vi "Test-XBox Controller-Request Updates.vi"() -> ()   [LabVIEW 2014, in "Comp XBox One Controller.lvlib"]
uses:
  Comp XBox One Controller.lvlib
  Robot Actor Framework/Trace/Trace Controller Class/Config.ctl
  Comp Motors with Encoders/Comp Motors with Encoders Class/Encoder Config.ctl
  Comp Motors with Encoders/Comp Motors with Encoders Class/Motor Controller Config.ctl
  Robot/Motor with Encoders/Motors with Encoders Class/Motors with Encoders Config.ctl
  Robot/Motor with Encoders/Motors with Encoders Class/Motors with Encoders State.ctl
  Comp Motors with Brake/Comp Motors with Brake Class/Comp Motors with Brake Config.ctl
  <vilib>/Rock Robotics/WPI/Solenoid/WPI_SolenoidChannel.ctl
  Comp Trace Controller/Comp Trace Controller Class/Comp Trace Controller.lvclass
  Comp Pressure/Comp Pressure Class/Comp Pressure.lvclass
  Comp Motors with Encoders/Receive Updates from Motors with Encoders Class/Receive Updates from Motors with Encoders.lvclass
  Comp Motors with Brake/Comp Motors with Brake Class/Comp Motors with Brake.lvclass
  <vilib>/Rock Robotics/WPI/DriverStation/WPI_DriverStationRobotMode2.ctl
  Comp Motors with Encoders/Receive Updates from Motors with Encoders Messages/Receive Update from Motors Msg/Receive Update from Motors Msg.lvclass
  Robot/Motor with Encoders/Motors with Encoders Messages/Request Motors with Encoders State Msg/Request Motors with Encoders State Msg.lvclass/Request Motors with Encoders State Msg.ctl
  <vilib>/ActorFramework/Message Enqueuer/Message Enqueuer.lvclass/Message Enqueuer.ctl
  Robot/Motor with Encoders/Motors with Encoders Messages/Set Rate (Percent) Msg/Set Rate (Percent) Msg.lvclass/Set Rate (Percent) Msg.ctl
  <vilib>/ActorFramework/Message Enqueuer/Enqueue.vi
  <vilib>/ActorFramework/Message Priority Queue/Priority Enqueue.vi
  Robot/Motor with Encoders/Motors with Encoders Messages/Request Motors with Encoders State Msg/Request Motors with Encoders State Msg.lvclass
  Robot/Motor with Encoders/Motors with Encoders Messages/Set Rate (Percent) Msg/Set Rate (Percent) Msg.lvclass
  <vilib>/ActorFramework/Stop Msg/Stop Msg.lvclass
  <vilib>/ActorFramework/Actor/Actor.lvclass
  Robot Actor Framework/Trace/Trace Controller Class/Trace Controller.lvclass
  Comp Motors with Encoders/Comp Motors with Encoders Class/Comp Motors with Encoders.lvclass
  Robot/Motor with Encoders/Motors with Encoders Class/Motors with Encoders.lvclass
panel:
  in  "Rate":dbl=0.5
  in  "Direction":enum32{"Up", "Hold", "Down"}(radio)
  in  "Comp Motors with Brake Config":T1={"Brake Channel"=enum."Solenoid 6", "Pneumatics CAN ID"=3}
  in  "Motors with Encoder State":T3={"Forward Switch"=FALSE, "Reverse Switch"=FALSE, "Measured RPM"=0.0, "Distance (in)"=0.0, "Setpoint RPM"=0.0, "Encoder Count"=0, "Home Count"=0, "Config"={"Counts  Per Revolution"=0, "Invert Encoder Direction"=FALSE, "Diameter of Revolution"=0.0, "Max RPM"=0.0, "Encoder Control"=TRUE}}
  in  "Motors with Encoders Config":T4={"Counts  Per Revolution"=256, "Invert Encoder Direction"=FALSE, "Diameter of Revolution"=1.5, "Max RPM"=500.0, "Encoder Control"=TRUE}
  in  "Slave Motor Controller Configs":T5[](array[typedef])
  in  "Master Motor Controller Config":T5={"Device Number"=7, "Invert Motor"=FALSE}
  in  "Encoder Config":T6={"P"=1.0, "D"=0.0, "F"=0.01, "I"=0.01, "Reverse Feedback Sensor"=FALSE, "Encoder Codes Per Rev"=256}
  in  "Test Loop":u32=75
  out "Enable Tele":bool caption="Enabled Teleop"
  in  "Stop Test Loop 1":bool=TRUE
  in  "Finish Test":bool=TRUE
  in  "Start Test":bool=TRUE
  in  "Trace Controller Config":T7={"Folder Pattern"="/media/sd%s1", "Starting Letter Position"=1, "Min Free Space (MB)"=50.0, "Max Folders to Check"=10, "Trace Level"=enum."Debug"} {"Min Free Space (MB)" format="%#_13g"}
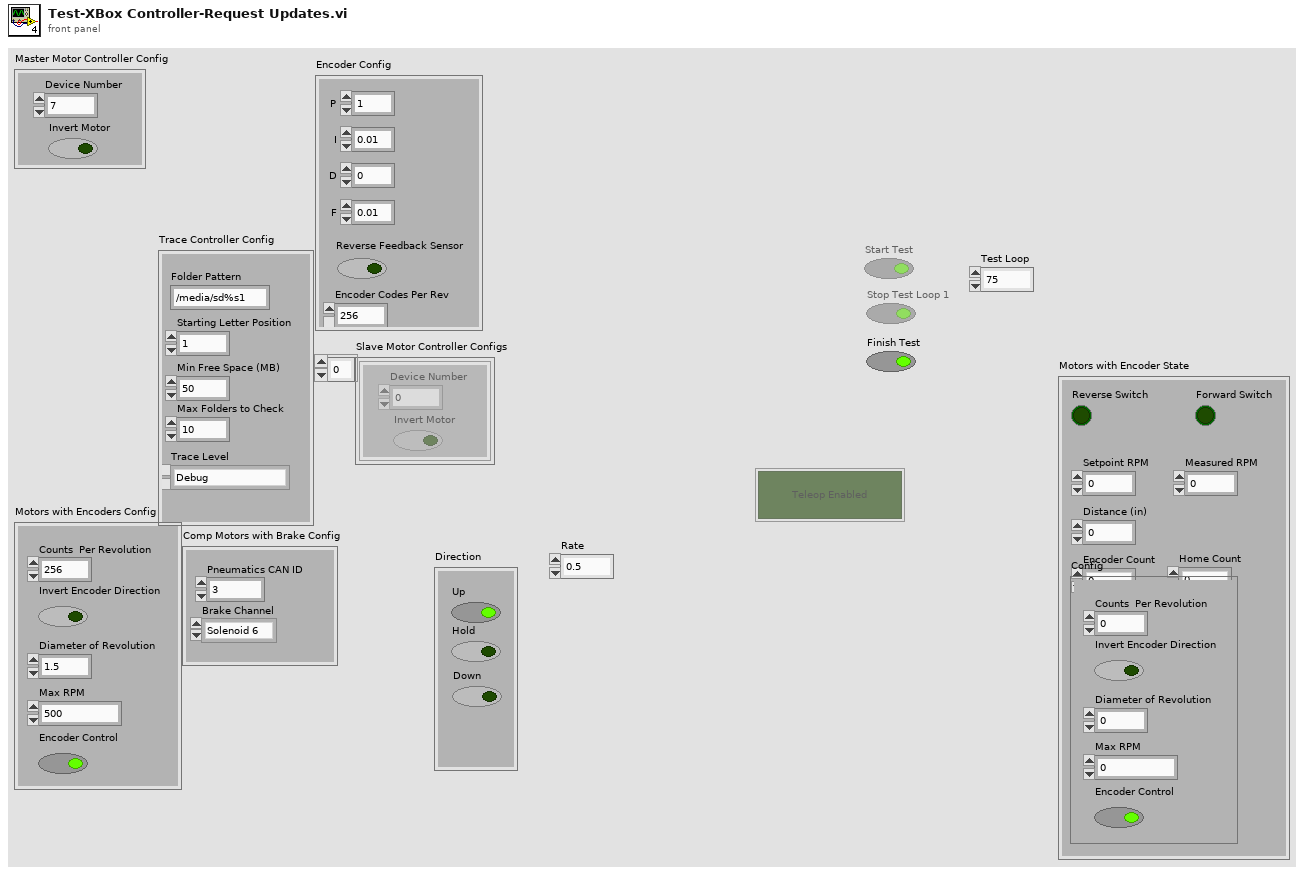
[diagram p1: front panel]
types:
  T1 = typedef "Comp Motors with Brake.lvlib/Comp Motors with Brake.lvclass/Comp Motors with Brake Config.ctl" = cluster{"Brake Channel":T2, "Pneumatics CAN ID":u8}
  T2 = typedef "WPI_SolenoidChannel.ctl" = enum8{"Solenoid 0", "Solenoid 1", "Solenoid 2", "Solenoid 3", "Solenoid 4", "Solenoid 5", "Solenoid 6", "Solenoid 7", "Invalid"}
  T3 = typedef "Motors with Encoders.lvlib/Motors with Encoders.lvclass/Motors with Encoders State.ctl" = cluster{"Forward Switch":bool, "Reverse Switch":bool, "Measured RPM":dbl, "Distance (in)":dbl, "Setpoint RPM":dbl, "Encoder Count":i64, "Home Count":i64, "Config":T4}
  T4 = typedef "Motors with Encoders.lvlib/Motors with Encoders.lvclass/Motors with Encoders Config.ctl" = cluster{"Counts  Per Revolution":u32, "Invert Encoder Direction":bool, "Diameter of Revolution":dbl, "Max RPM":dbl, "Encoder Control":bool}
  T5 = typedef "Comp Motors with Encoders.lvlib/Comp Motors with Encoders.lvclass/Motor Controller Config.ctl" = cluster{"Device Number":u8, "Invert Motor":bool}
  T6 = typedef "Comp Motors with Encoders.lvlib/Comp Motors with Encoders.lvclass/Encoder Config.ctl" = cluster{"P":dbl, "D":dbl, "F":dbl, "I":dbl, "Reverse Feedback Sensor":bool, "Encoder Codes Per Rev":u16}
  T7 = typedef "Robot Actor Framework.lvlib/Trace.lvlib/Trace Controller.lvclass/Config.ctl" = cluster{"Folder Pattern":string, "Starting Letter Position":i32, "Min Free Space (MB)":dbl, "Max Folders to Check":u32, "Trace Level":enum16{"Critical", "Error", "Warning", "Informational", "Debug"}}
  T8 = enum16{"Critical", "Error", "Warning", "Informational", "Debug"}
  T9 = enum8{"Enabled", "Disabled", "Disabled and Grayed Out"}
  T10 = typedef "WPI_DriverStationRobotMode2.ctl" = enum16{"Autonomous Disabled", "Autonomous Enabled", "Teleop Disabled", "Teleop Enabled", "Disconnected", "Finish", "Test Disabled", "Test Enabled", "Emergency Stopped"}
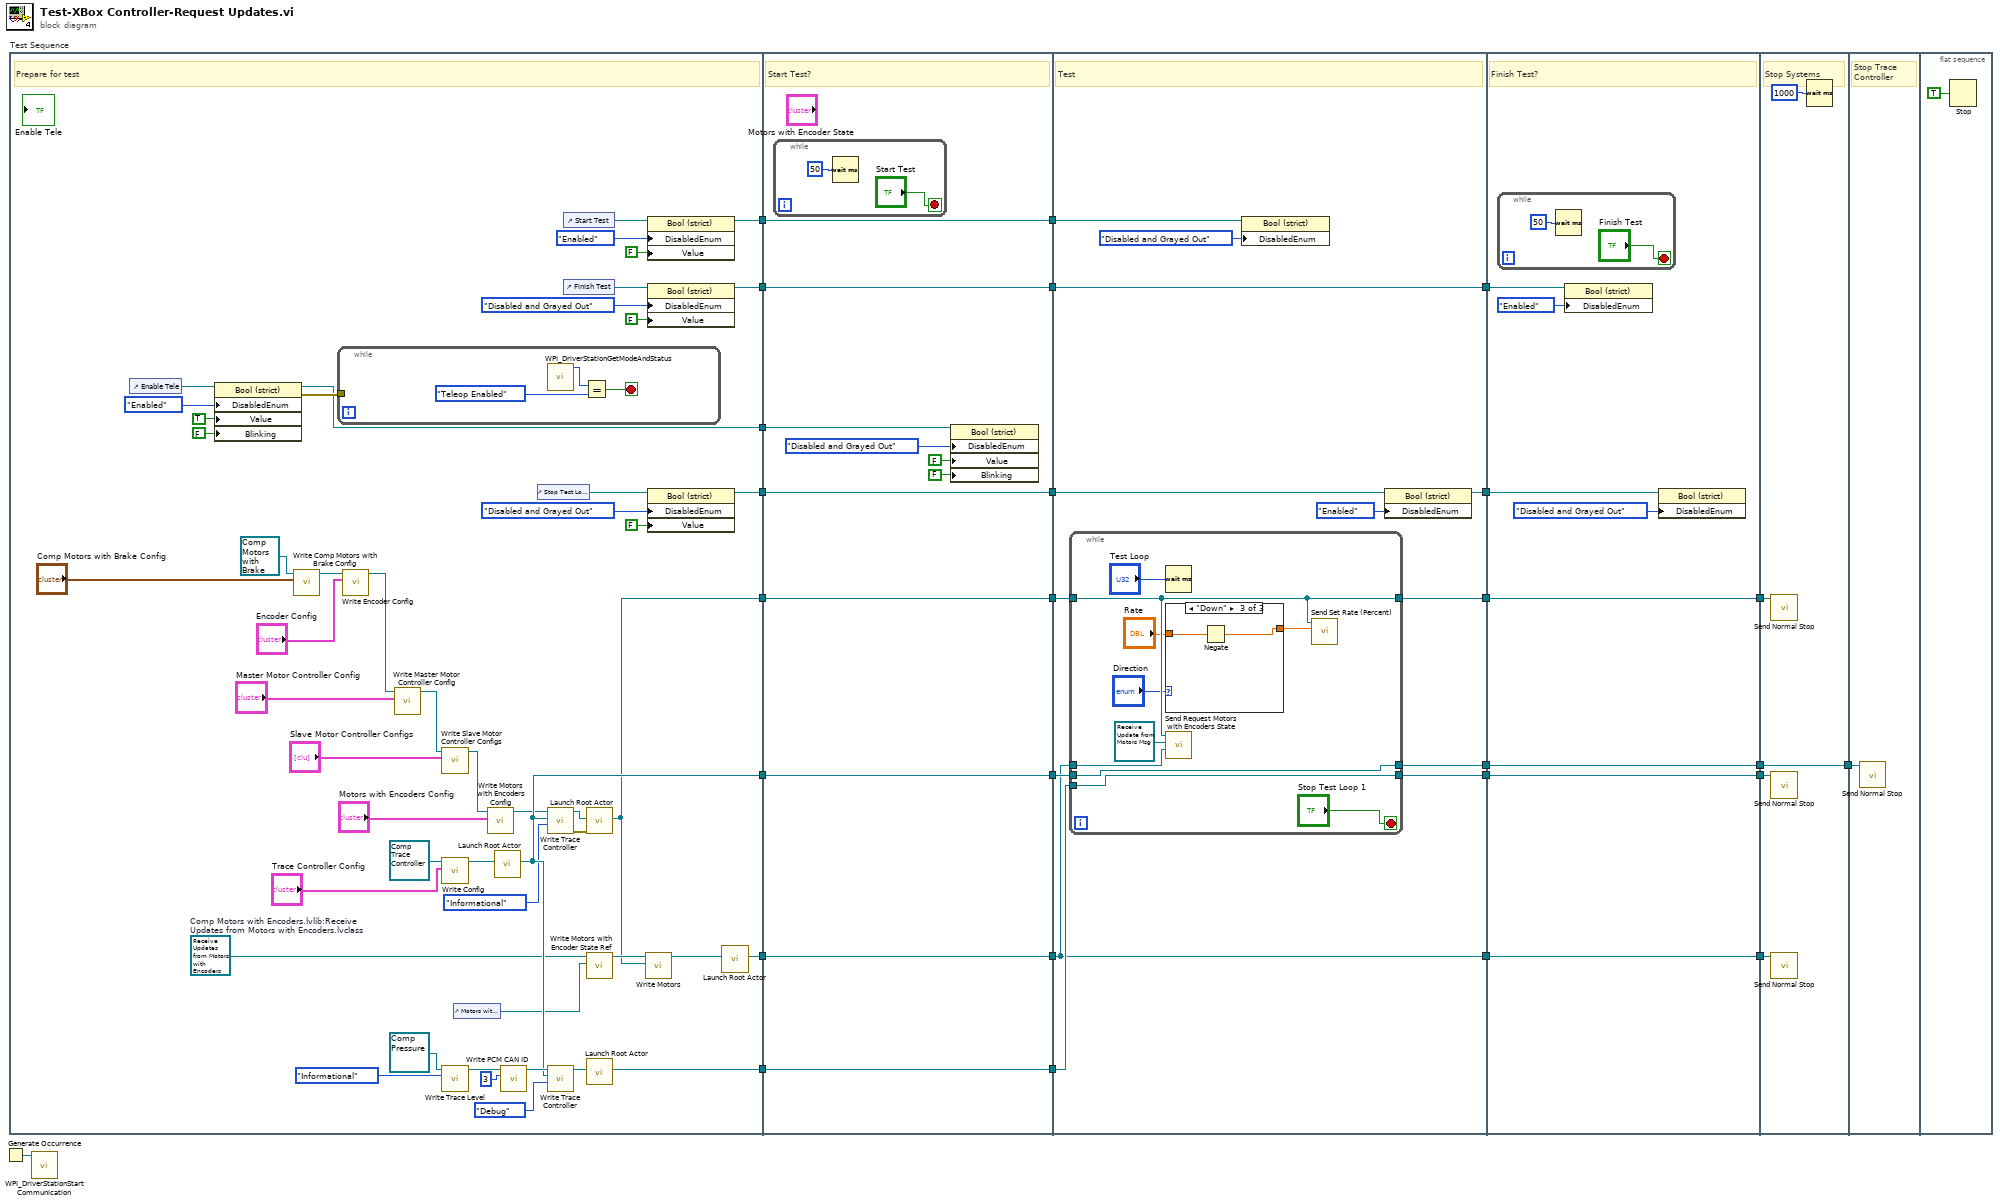
[diagram p0: block diagram]
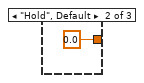
[diagram p3: hidden frame]
diagram:
  n1 = Generate Occurrence() -> (w27:refnum<k4>)
  n2 = flat-sequence "Test Sequence" {
    tunnel: [w32] -> w16
    tunnel: [w67] -> w15
    tunnel: [w66] -> w14
    tunnel: [w56] -> w13
    tunnel: [w55] -> w11
    tunnel: [w54] -> w6
    tunnel: [w48] -> w5
    tunnel: [w45] -> w3
    tunnel: [w91] -> w19
    tunnel: [w90] -> w18
    tunnel: [w89] -> w17
    tunnel: w16 -> [w91]
    tunnel: w15 -> [w90]
    tunnel: w14 -> [w89]
    tunnel: w13 -> [w88]
    tunnel: [w88] -> w12
    tunnel: w11 -> [w87]
    tunnel: [w87] -> w10
    tunnel: [w86] -> w7
    tunnel: w6 -> [w86]
    tunnel: w5 -> [w85]
    tunnel: [w81] -> w4
    tunnel: w3 -> [w81]
    tunnel: [w101] -> w22
    tunnel: [w103] -> w21
    tunnel: [w102] -> w20
    tunnel: w19 -> [w106]
    tunnel: w18 -> [w104]
    tunnel: w17 -> [w105]
    tunnel: w12 -> [w100]
    tunnel: w10 -> [w98]
    tunnel: [w96] -> w9
    tunnel: [w95] -> w8
    tunnel: w7 -> [w95]
    tunnel: w4 -> [w94]
    tunnel: [w94] -> w2
    tunnel: [w128] -> w25
    tunnel: [w127] -> w24
    tunnel: [w126] -> w23
    tunnel: w22 -> [w128]
    tunnel: w21 -> [w127]
    tunnel: w20 -> [w126]
    tunnel: w9 -> [w125]
    tunnel: w8 -> [w122]
    tunnel: w2 -> [w121]
    tunnel: [w121] -> w1
    tunnel: [w135] -> w26
    tunnel: w25 -> [w135]
    tunnel: w24 -> [w134]
    tunnel: w23 -> [w132]
    tunnel: w1 -> [w131]
    tunnel: w26 -> [w136]
    frame #0 {
      w35 = refnum<class "Receive Updates from Motors with Encoders.lvclass"> refnum  # Comp Motors with Encoders.lvlib:Receive Updates from Motors with Encoders.lvclass
      # "Prepare for test"
      n3 = control-ref of="Enable Tele"() -> (w53:refnum<vi>)
      n4 = property class="Bool (strict)"(reference=w53, "DisabledEnum"=T9."Enabled" ("Disabled"), "Value"=TRUE, "Blinking"=FALSE) -> (reference out=w48:refnum<vi>, error out=w50:errorcluster)  [unwired: 1 in]
      n5 = call-dynamic "Write Comp Motors with Brake Config.vi"("Comp Motors with Brake Config"="Comp Motors with Brake Config", "Comp Motors with Brake in"=refnum<class "Comp Motors with Brake.lvclass"> refnum ("Comp Motors with Brake.lvlib:Comp Motors with Brake.lvclass")) -> ("Comp Motors with Brake out"=w29:refnum<class "Comp Motors with Brake.lvclass">)  [unwired: 8 in, 1 out]
      n6 = while {
        tunnel: w50 -> [_]
        stop <- w78 stop-if-true
        n7 = call <vilib>:"WPI_DriverStationGetModeAndStatus.vi"() -> ("Robot Mode"=w80:T10)  [unwired: 10 in, 1 out]
        n8 = Equal?(x=w80, y=WPI_DriverStationRobotMode2."Teleop Enabled") -> (x = y?=w78:bool)
      }
      n9 = call-dynamic "Write Encoder Config.vi"("Encoder Config"="Encoder Config", "Comp Motors with Encoders in"=w29) -> ("Comp Motors with Encoders out"=w43:refnum<class "Comp Motors with Brake.lvclass">)  [unwired: 8 in, 1 out]
      n10 = call-dynamic "Write Master Motor Controller Config.vi"("Master Motor Controller Config"="Master Motor Controller Config", "Comp Motors with Encoders in"=w43) -> ("Comp Motors with Encoders out"=w42:refnum<class "Comp Motors with Brake.lvclass">)  [unwired: 8 in, 1 out]
      n11 = call-dynamic "Write Slave Motor Controller Configs.vi"("Slave Motor Controller Configs"="Slave Motor Controller Configs", "Comp Motors with Encoders in"=w42) -> ("Comp Motors with Encoders out"=w41:refnum<class "Comp Motors with Brake.lvclass">)  [unwired: 8 in, 1 out]
      n12 = call-dynamic "Write Config.vi"("Config"="Trace Controller Config", "Trace Controller in"=refnum<class "Comp Trace Controller.lvclass"> refnum ("Comp Trace Controller.lvlib:Comp Trace Controller.lvclass")) -> ("Trace Controller out"=w70:refnum<class "Comp Trace Controller.lvclass">)  [unwired: 8 in, 1 out]
      n13 = call-dynamic "Write Trace Level.vi"("Trace Level"=T8."Informational", "System Actor in"=refnum<class "Comp Pressure.lvclass"> refnum ("Comp Pressure.lvlib:Comp Pressure.lvclass")) -> ("System Actor out"=w75:refnum<class "Comp Pressure.lvclass">)  [unwired: 8 in, 1 out]
      n14 = control-ref of="Motors with Encoder State"() -> (w34:refnum<vi>)
      n15 = call-dynamic "Write Motors with Encoders Config.vi"("Motors with Encoders Config"="Motors with Encoders Config", "Motors with Encoders in"=w41) -> ("Motors with Encoders out"=w36:refnum<class "Comp Motors with Brake.lvclass">)  [unwired: 8 in, 1 out]
      n16 = call <vilib>:"Launch Root Actor.vi"("Actor"=w70) -> ("Actor's Enqueuer"=w66:refnum<class "Message Enqueuer.lvclass">)  [unwired: 9 in, 1 out]
      n17 = call-dynamic "Write PCM CAN ID.vi"("PCM CAN ID"=u8 3, "Comp Pressure in"=w75) -> ("Comp Pressure out"=w76:refnum<class "Comp Pressure.lvclass">)  [unwired: 8 in, 1 out]
      n18 = control-ref of="Stop Test Loop 1"() -> (w60:refnum<vi>)
      n19 = call-dynamic "Write Trace Controller.vi"("Trace Level"=T8."Informational", "Trace Controller"=w66, "System Actor in"=w36) -> ("error out"=w72:errorcluster, "System Actor out"=w71:refnum<class "Comp Motors with Brake.lvclass">)  [unwired: 7 in]
      n20 = call-dynamic "Write Trace Controller.vi"("Trace Level"=T8."Debug", "Trace Controller"=w66, "System Actor in"=w76) -> ("System Actor out"=w77:refnum<class "Comp Pressure.lvclass">)  [unwired: 7 in, 1 out]
      n21 = control-ref of="Start Test"() -> (w65:refnum<vi>)
      n22 = control-ref of="Finish Test"() -> (w59:refnum<vi>)
      n23 = call <vilib>:"Launch Root Actor.vi"("error in (no error)"=w72, "Actor"=w71) -> ("Actor's Enqueuer"=w32:refnum<class "Message Enqueuer.lvclass">)  [unwired: 8 in, 1 out]
      n24 = call-dynamic "Write Motors with Encoder State Ref.vi"("Motors with Encoder State Ref"=w34, "Receive Updates from Motors with Encoders in"=w35) -> ("Receive Updates from Motors with Encoders out"=w33:refnum<class "Receive Updates from Motors with Encoders.lvclass">)  [unwired: 8 in, 1 out]
      n25 = call <vilib>:"Launch Root Actor.vi"("Actor"=w77) -> ("Actor's Enqueuer"=w67:refnum<class "Message Enqueuer.lvclass">)  [unwired: 9 in, 1 out]
      n26 = call-dynamic "Write Motors.vi"("Actor Framework:Message Enqueuer"=w32, "Receive Updates from Motors with Encoders in"=w33) -> ("Receive Updates from Motors with Encoders out"=w31:refnum<class "Receive Updates from Motors with Encoders.lvclass">)  [unwired: 8 in, 1 out]
      n27 = property class="Bool (strict)"(reference=w65, "DisabledEnum"=T9."Enabled" ("Disabled"), "Value"=FALSE) -> (reference out=w56:refnum<vi>)  [unwired: 1 in, 1 out]
      n28 = property class="Bool (strict)"(reference=w59, "DisabledEnum"=T9."Disabled and Grayed Out" ("Disabled"), "Value"=FALSE) -> (reference out=w54:refnum<vi>)  [unwired: 1 in, 1 out]
      n29 = property class="Bool (strict)"(reference=w60, "DisabledEnum"=T9."Disabled and Grayed Out" ("Disabled"), "Value"=FALSE) -> (reference out=w55:refnum<vi>)  [unwired: 1 in, 1 out]
      n30 = call <vilib>:"Launch Root Actor.vi"("Actor"=w31) -> ("Actor's Enqueuer"=w45:refnum<class "Message Enqueuer.lvclass">)  [unwired: 9 in, 1 out]
    }
    frame #1 {
      # "Start Test?"
      n31 = while {
        stop <- "Start Test" stop-if-true
        n32 = Wait (ms)(milliseconds to wait=u32 50) -> ()  [unwired: 1 out]
      }
      n33 = property class="Bool (strict)"(reference=w85, "DisabledEnum"=T9."Disabled and Grayed Out" ("Disabled"), "Value"=FALSE, "Blinking"=FALSE) -> ()  [unwired: 1 in, 2 out]
    }
    frame #2 {
      # "Test"
      n34 = while {
        tunnel: w105 -> [w115]
        tunnel: [w115] -> w101
        tunnel: w106 -> [w110]
        tunnel: [w110] -> w103
        tunnel: w104 -> [w114]
        tunnel: [w114] -> w102
        tunnel: w94 -> [w112]
        stop <- "Stop Test Loop 1" stop-if-true
        n35 = Wait (ms)(milliseconds to wait="Test Loop") -> ()  [unwired: 1 out]
        n36 = case shown="\"Down\"" "Direction" {
          tunnel: [w117 0.0 w119] -> w108
          tunnel: "Rate" -> [w117 _ w120]
          frame "Up" {
          }
          frame "Hold", Default {
          }
          frame "Down" {
            n37 = Negate(x=w120) -> (-x=w119:dbl)
          }
        }
        n38 = call "Send Request Motors with Encoders State.vi"("Requestor Queue"=w112, "Current State Msg"=refnum<class "Receive Update from Motors Msg.lvclass"> refnum ("Comp Motors with Encoders.lvlib:Receive Update from Motors Msg.lvclass"), "Message Enqueuer"=w110) -> ()  [unwired: 7 in, 2 out]
        n39 = call "Send Set Rate (Percent).vi"("Rate (Percentage)"=w108, "Message Enqueuer"=w110) -> ()  [unwired: 8 in, 2 out]
      }
      n40 = property class="Bool (strict)"(reference=w100, "DisabledEnum"=T9."Disabled and Grayed Out" ("Disabled")) -> ()  [unwired: 1 in, 2 out]
      n41 = property class="Bool (strict)"(reference=w98, "DisabledEnum"=T9."Enabled" ("Disabled")) -> (reference out=w96:refnum<vi>)  [unwired: 1 in, 1 out]
    }
    frame #3 {
      # "Finish Test?"
      n42 = while {
        stop <- "Finish Test" stop-if-true
        n43 = Wait (ms)(milliseconds to wait=u32 50) -> ()  [unwired: 1 out]
      }
      n44 = property class="Bool (strict)"(reference=w122, "DisabledEnum"=T9."Enabled" ("Disabled")) -> ()  [unwired: 1 in, 2 out]
      n45 = property class="Bool (strict)"(reference=w125, "DisabledEnum"=T9."Disabled and Grayed Out" ("Disabled")) -> ()  [unwired: 1 in, 2 out]
    }
    frame #4 {
      # "Stop Systems"
      n46 = call <vilib>:"Send Normal Stop.vi"("Message Enqueuer"=w134) -> ()  [unwired: 10 in, 1 out]
      n47 = call <vilib>:"Send Normal Stop.vi"("Message Enqueuer"=w132) -> ()  [unwired: 10 in, 1 out]
      n48 = call <vilib>:"Send Normal Stop.vi"("Message Enqueuer"=w131) -> ()  [unwired: 10 in, 1 out]
      n49 = Wait (ms)(milliseconds to wait=u32 1000) -> ()  [unwired: 1 out]
    }
    frame #5 {
      # "Stop Trace Controller"
      n50 = call <vilib>:"Send Normal Stop.vi"("Message Enqueuer"=w136) -> ()  [unwired: 10 in, 1 out]
    }
    frame #6 {
      n51 = Stop(stop? (T)=TRUE) -> ()
    }
  }
  n52 = call <vilib>:"WPI_DriverStationStart Communication.vi"("occurrence"=w27) -> ()  [unwired: 1 in, 10 out]
